vi "USB2XXXGPIOTest.vi"() -> ()   [LabVIEW 2010]
panel:
  in  "stop":bool
  out "P15":bool
  out "P14":bool
  out "P13":bool
  out "P12":bool
  out "P11":bool
  out "P10":bool
  out "P9":bool
  out "P8":bool
  in  "P7":bool
  in  "P6":bool
  in  "P5":bool
  in  "P4":bool
  in  "P3":bool
  in  "P2":bool
  in  "P1":bool
  in  "P0":bool
  in  "Device Index":i32(ring) items=["0", "1", "2", "3", "4", "5"]
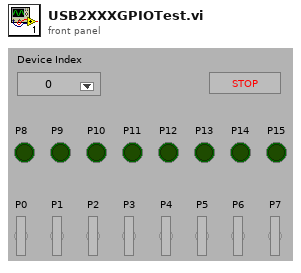
[diagram p1: front panel]
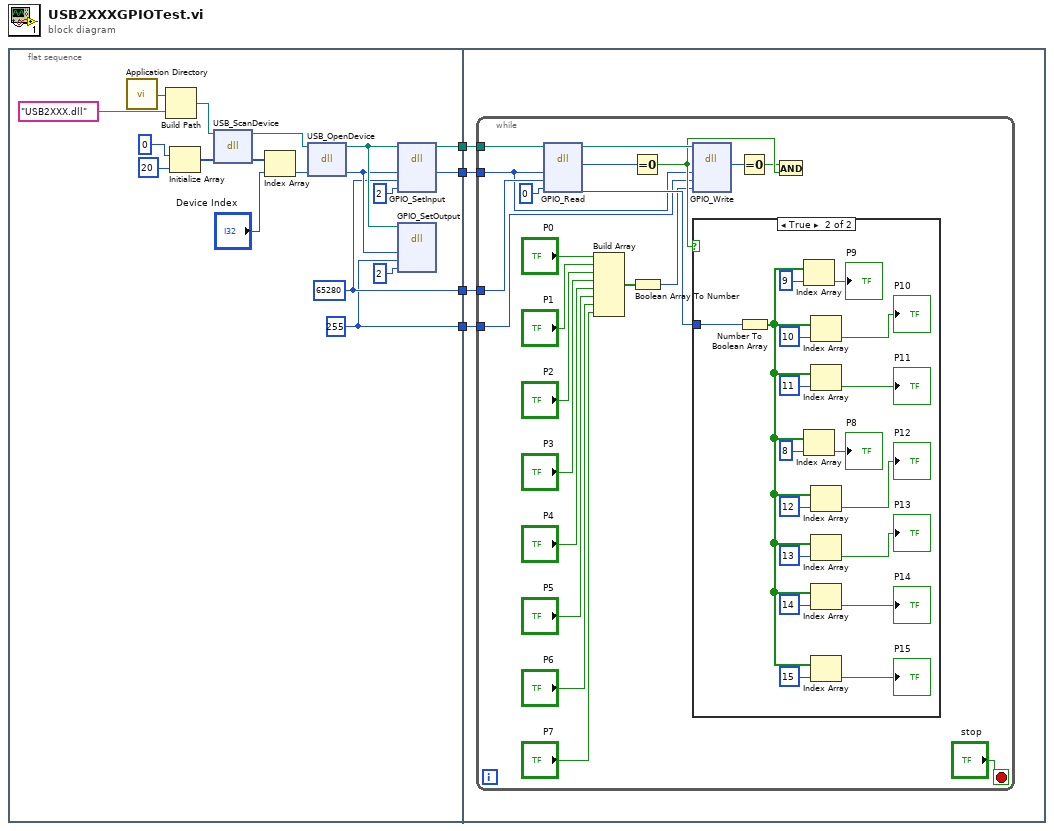
[diagram p0: block diagram]
diagram:
  n1 = flat-sequence {
    tunnel: [w8] -> w4
    tunnel: [w7] -> w3
    tunnel: [w6] -> w2
    tunnel: [w5] -> w1
    tunnel: w4 -> [w26]
    tunnel: w3 -> [w25]
    tunnel: w2 -> [w24]
    tunnel: w1 -> [w23]
    frame #0 {
      w6 = u32 65280
      w5 = u32 255
      n2 = call <vilib>:"Application Directory.vi"() -> ("Application Directory"=w22:path)
      n3 = Build Path(base path=w22, name or relative path="USB2XXX.dll") -> (appended path=w15:path)
      n4 = Initialize Array(0, 20 ("dimension size")) -> (w16:i32[])
      n5 = dll-call lib="E:/OtherWork/STM32/USB2XXX_Example/trunk/Labview/PublicFiles/USB2XXX.*" fn="USB_ScanDevice"(path in=w15, "pDevNum"=w16) -> (path out=w14:path, "pDevNum"=w19:i32[])  [unwired: 3 in, 1 out]
      n6 = Index Array(array=w19, index="Device Index") -> (element=w13:i32)
      n7 = dll-call lib="E:/OtherWork/STM32/USB2XXX_Example/trunk/Labview/PublicFiles/USB2XXX.*" fn="USB_OpenDevice"(path in=w14, "DevIndex"=w13) -> (path out=w10:path, "DevIndex"=w9:i32)  [unwired: 3 in, 1 out]
      n8 = dll-call lib="E:/OtherWork/STM32/USB2XXX_Example/trunk/Labview/PublicFiles/USB2XXX.*" fn="GPIO_SetInput"(path in=w10, "DevHandle"=w9, "PinMask"=w6, "PuPd"=u8 2) -> (path out=w8:path, "DevHandle"=w7:i32)  [unwired: 5 in, 1 out]
      n9 = dll-call lib="E:/OtherWork/STM32/USB2XXX_Example/trunk/Labview/PublicFiles/USB2XXX.*" fn="GPIO_SetOutput"(path in=w10, "DevIndex"=w9, "PinMask"=w5, "PuPd"=u8 2) -> ()  [unwired: 6 in, 2 out]
    }
    frame #1 {
      n10 = while {
        tunnel: w26 -> [w30]
        tunnel: w25 -> [w28]
        tunnel: w24 -> [w29]
        tunnel: w23 -> [w27]
        stop <- "stop" stop-if-true
        n11 = dll-call lib="E:/OtherWork/STM32/USB2XXX_Example/trunk/Labview/PublicFiles/USB2XXX.*" fn="GPIO_Read"(path in=w30, "DevIndex"=w28, "PinMask"=w29, "pPinValue"=u32 0) -> (path out=w47:path, "return type"=w42:i32, "pPinValue"=w43:u32)  [unwired: 4 in, 1 out]
        n12 = Build Array("P0", "P1", "P2", "P3", "P4", "P5", "P6", "P7") -> (w39:bool[])
        n13 = Equal To 0?(x=w42) -> (x = 0?=w46:bool)
        n14 = Boolean Array To Number(Boolean array=w39) -> (number=w40:u32)
        n15 = dll-call lib="E:/OtherWork/STM32/USB2XXX_Example/trunk/Labview/PublicFiles/USB2XXX.*" fn="GPIO_Write"(path in=w47, "DevIndex"=w28, "PinMask"=w27, "PinValue"=w40) -> ("return type"=w44:i32)  [unwired: 5 in, 2 out]
        n16 = case shown="True" w46 {
          tunnel: w43 -> [_ w66]
          frame False {
          }
          frame True {
            n17 = Number To Boolean Array(number=w66) -> (Boolean array=w56:bool[])
            n18 = Index Array(array=w56, index=9) -> (element=→"P9":bool)
            n19 = Index Array(array=w56, index=8) -> (element=→"P8":bool)
            n20 = Index Array(array=w56, index=10) -> (element=→"P10":bool)
            n21 = Index Array(array=w56, index=11) -> (element=→"P11":bool)
            n22 = Index Array(array=w56, index=12) -> (element=→"P12":bool)
            n23 = Index Array(array=w56, index=13) -> (element=→"P13":bool)
            n24 = Index Array(array=w56, index=14) -> (element=→"P14":bool)
            n25 = Index Array(array=w56, index=15) -> (element=→"P15":bool)
          }
        }
        n26 = Equal To 0?(x=w44) -> (x = 0?=w45:bool)
        n27 = And(x=w45, y=w46) -> ()  [unwired: 1 out]
      }
    }
  }
